vi "Stop.vi"(8 "error in (no error)":errorcluster, 11 "LabBOT in":refnum<class "LabBOT.lvclass">) -> (0 "error out":errorcluster, 3 "LabBOT out":refnum<class "LabBOT.lvclass">)   [LabVIEW 2020, in "Rover.lvlib" / "LabBOT.lvclass"]
uses:
  LabBOT.lvclass
  LabBOT.lvclass/LabBOT.ctl
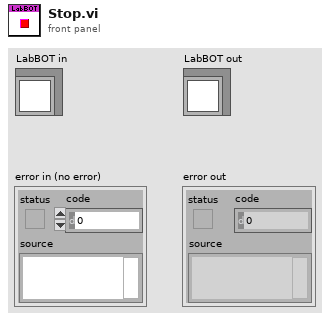
[diagram p1: front panel]
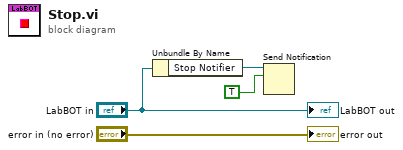
[diagram p0: block diagram]
diagram:
  n1 = Unbundle By Name("LabBOT in") -> ("Stop Notifier"=w2:refnum<notifier>)
  n2 = Send Notification(notification=TRUE, notifier=w2) -> ()  [unwired: 1 in, 2 out]
  "error out" <- "error in (no error)"
  "LabBOT out" <- "LabBOT in"
